vi "Calculate Total Time.vi"(10 "Boolean array":bool[](array[boolean]), 11 "FP":T1) -> (3 "Total Time(s)":dbl)   [LabVIEW 2020]
uses:
  Main Refs.ctl
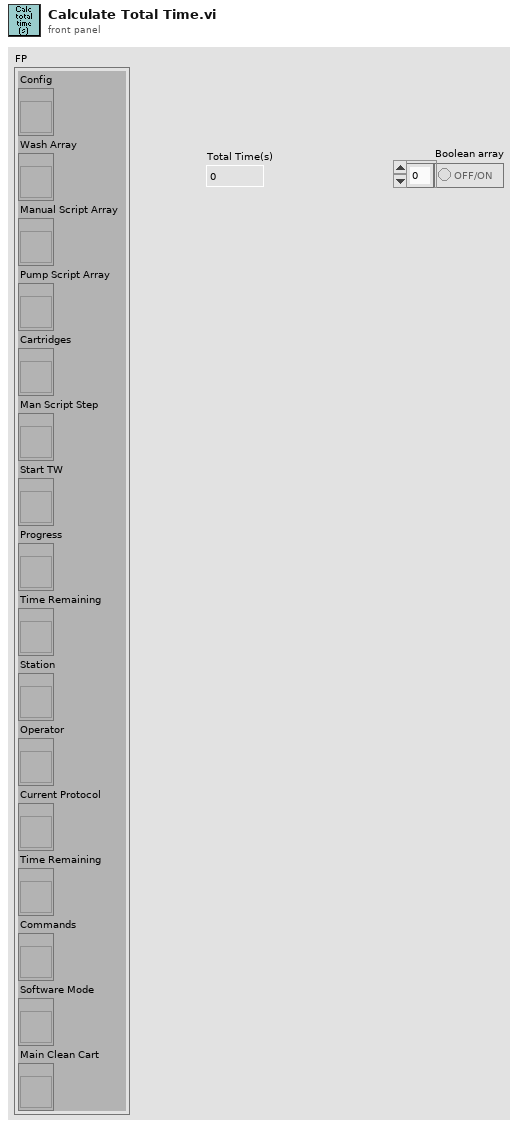
[diagram p1: front panel]
types:
  T1 = typedef "Main Refs.ctl" = cluster{"Config":refnum<vi>, "Wash Array":refnum<vi>, "Manual Script Array":refnum<vi>, "Pump Script Array":refnum<vi>, "Cartridges":refnum<vi>, "Man Script Step":refnum<vi>, "Start TW":refnum<vi>, "Progress":refnum<vi>, "Time Remaining":refnum<vi>, "Station":refnum<vi>, "Operator":refnum<vi>, "Current Protocol":refnum<vi>, "Time Remaining":refnum<vi>, "Commands":refnum<vi>, "Software Mode":refnum<vi>, "Main Clean Cart":refnum<vi>}
  T2 = typedef "Pump Config.ctl" = cluster{"Syringe size":u32, "Syringe address":u32, "# of ports":u32, "Init String":string, "Full Stroke (cnts)":i32, "Model":enum16{"XC", "Centris"}, "TW Position":dbl, "Load Position":dbl, "Bottom Position":dbl, "Station ID":string, "Default Protocol":path, "Dry Time(s)":dbl, "Python Version":string, "NFC SN Array":string[], "Timing":T3, "Pressure Specs":T4}
  T3 = typedef "Timing Specs.ctl" = cluster{"Checking pres and leak":dbl, "Priming input lines":dbl, "Rinsing syringe":dbl, "Filling well X w/ X":dbl, "Drain well X":dbl, "Clearing wells and lines":dbl, "Draining wells":dbl, "Rinsing all wells":dbl, "Testing for leaks/clogs":dbl, "Rinsing wells":dbl}
  T4 = typedef "Vacuum Specs.ctl" = cluster{"Pressure max":dbl, "Pressure min":dbl, "Decay delta":dbl, "Pressure time":dbl, "Conf. R":dbl, "LeakRateMax":dbl}
  T5 = typedef "Wash Step.ctl" = cluster{"Reagent":string, "Bottle":enum16{"Bottle 1", "Bottle 2", "Bottle 3", "Bottle 4"}, "Wash Time(s)":dbl, "Dwell Time(s)":dbl, "# of Rinses":i16}
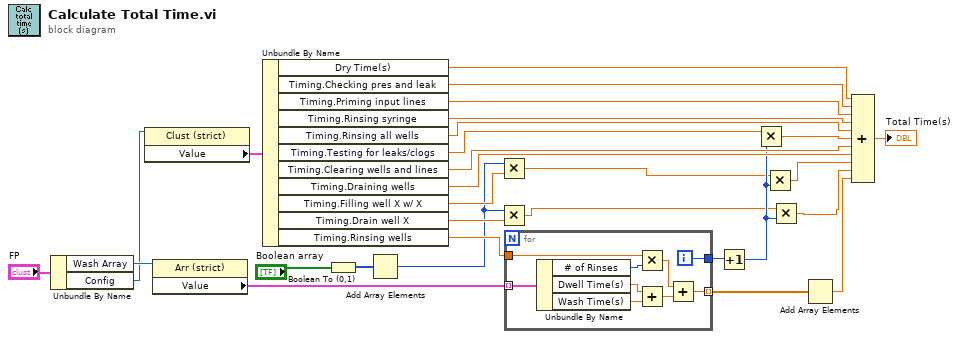
[diagram p0: block diagram]
diagram:
  n1 = Unbundle By Name("FP") -> ("Wash Array"=w29:refnum<vi>, "Config"=w25:refnum<vi>)
  n2 = property class="Clust (strict)"(reference=w25) -> ("Value"=w24:T2)  [unwired: 1 in, 2 out]
  n3 = property class="Arr (strict)"(reference=w29) -> ("Value"=w26:T5[])  [unwired: 1 in, 2 out]
  n4 = Unbundle By Name(w24) -> ("Dry Time(s)"=w23:dbl, "Timing.Checking pres and leak"=w22:dbl, "Timing.Priming input lines"=w21:dbl, "Timing.Rinsing syringe"=w20:dbl, "Timing.Rinsing all wells"=w16:dbl, "Timing.Testing for leaks/clogs"=w10:dbl, "Timing.Clearing wells and lines"=w19:dbl, "Timing.Draining wells"=w18:dbl, "Timing.Filling well X w/ X"=w15:dbl, "Timing.Drain well X"=w14:dbl, "Timing.Rinsing wells"=w17:dbl)
  n5 = Boolean To (0,1)(Boolean="Boolean array") -> (0, 1=w7:i16[])
  n6 = Add Array Elements(numeric array=w7) -> (sum=w6:i16)
  n7 = Multiply(x=w6, y=w15) -> (x*y=w4:dbl)
  n8 = Multiply(x=w6, y=w14) -> (x*y=w3:dbl)
  n9 = for {
    tunnel: w26 -> [w38] mode=indexing
    tunnel: [w37] -> w28 mode=indexing
    tunnel: w17 -> [w31]
    tunnel: [w30] -> w9
    i -> [w30]
    n10 = Unbundle By Name(w38) -> ("# of Rinses"=w32:i16, "Dwell Time(s)"=w34:dbl, "Wash Time(s)"=w35:dbl)
    n11 = Multiply(x=w31, y=w32) -> (x*y=w33:dbl)
    n12 = Add(x=w34, y=w35) -> (x+y=w36:dbl)
    n13 = Add(x=w33, y=w36) -> (x+y=w37:dbl)
  }
  n14 = Increment(x=w9) -> (x+1=w5:i32)
  n15 = Multiply(x=w10, y=w5) -> (x*y=w11:dbl)
  n16 = Multiply(x=w4, y=w5) -> (x*y=w1:dbl)
  n17 = Multiply(x=w3, y=w5) -> (x*y=w2:dbl)
  n18 = Add Array Elements(numeric array=w28) -> (sum=w13:dbl)
  n19 = Compound Arithmetic op=ADD(w23, w22, w21, w20, w16, w11, w19, w18, w1, w2, w13) -> (→"Total Time(s)":dbl)
